vi "HXG2_NPSH Calc.vi"() -> ()   [LabVIEW 2012]
panel:
  in  "Pump dP (psid)":dbl
  in  "P atm (psi)":dbl
  in  "Pump Pressure (psig)":dbl
  out "error out":errorcluster
  in  "error in (no error)":errorcluster
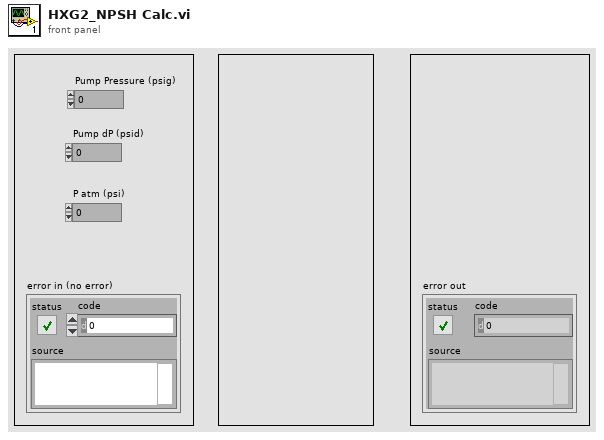
[diagram p1: front panel]
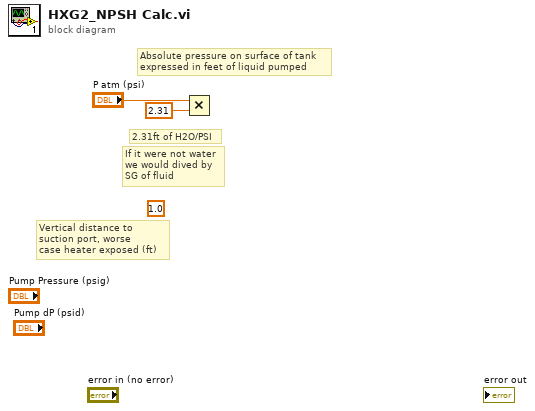
[diagram p0: block diagram]
diagram:
  (unwired) 1.0 ("y")
  # "Vertical distance to suction port, worse\ncase heater exposed (ft)"
  # "If it were not water\nwe would dived by\nSG of fluid"
  # "2.31ft of H2O/PSI"
  # "Absolute pressure on surface of tank\nexpressed in feet of liquid pumped"
  n1 = Multiply(x="P atm (psi)", y=2.31) -> ()  [unwired: 1 out]
